vi "ReadWrite.vi"(4 "read":bool=TRUE, 5 "delay before read (ms)":u32=50, 6 "error in":errorcluster, 7 "write":bool=TRUE, 8 "string to write":string="*IDN?\r\n", 9 "VISA  name in":refnum<visa-resource-name>) -> (0 "error out":errorcluster, 1 "bytes to read":u32, 2 "read string":string, 3 "VISA out":refnum<visa-resource-name>)   [LabVIEW 2017]
doc: "The Basic Serial Read and Write example performs a Serial Port Read, a Serial Port Write, or a combination of these actions. The user selects the actions (read or write) on the front panel. If both are selected, the VI will write the data first, read data, and then close the VISA session that is opened to the port. This VI will wait until the specified number of bytes is received at the port. Only the number of bytes specified will be read.\n\nINSTRUCTIONS:\n1) Select the serial resource and configuration parameters (baud rate, data bits, parity, stop bits, flow control).\n2) Select the operations to be performed. \n3) Connect the serial port to your device. If no device is available, perform a loopback test by doing one of the following. Short pins 2 and 3 on a RS-232 cable or short pin 4 to pin 8 and pin 5 to pin 9 on a RS-485/422 cable. \n4) Run the VI to see the data read. (The \"read string\" will match the \"string to write\" if a loopback test was performed.)\n\nNote: The parameters set for the serial port must match the parameters of the connected instrument or device. In this example, the bytes to read parameter specifies the number of bytes that the serial port reads. If there were more bytes at the port than the number specified in bytes to read, those bytes would not be read. Also, if you specify to read more bytes than the number of bytes actually read, you might receive a timeout error message.\n\nOn the block diagram, the Configure Serial Port VI sets the configuration parameters. The front panel displays the controls used to configure the basic parameters, such as baud rate, data bits, and parity. Constants configure the other parameters the user probably does not need set. After the VISA Configure Serial Port VI opens the VISA session and configures the port, the VI passes the VISA resource name to other VIs that perform operations on that VISA resource. The VISA Write function sends a command to the serial device and the VISA Read function returns data based on the command. The VISA Close function then closes the reference to the serial device. It is important to close the reference; otherwise communication through with that port through protocols other than VISA might not be possible."
panel:
  out "bytes read":u32
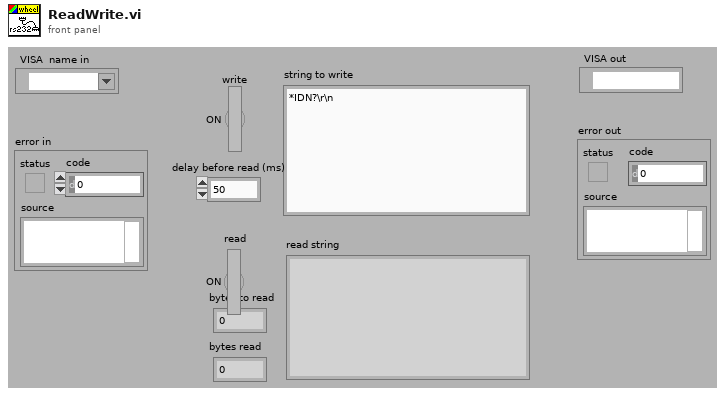
[diagram p1: front panel]
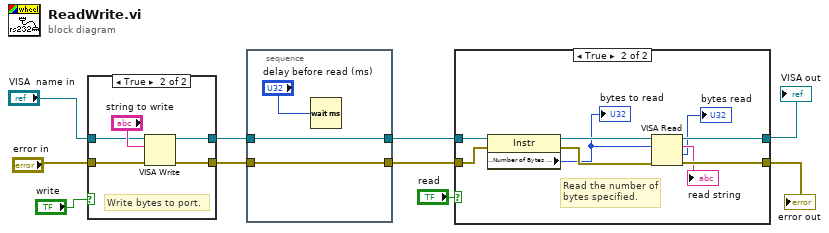
[diagram p0: block diagram]
diagram:
  n1 = case shown="True" "write" {
    tunnel: [w12 w17] -> w6
    tunnel: "VISA  name in" -> [w11 w15]
    tunnel: "error in" -> [w12 w14]
    tunnel: [w11 w13] -> w4
    frame False {
    }
    frame True {
      # "Write bytes to port."
      n2 = VISA Write(VISA resource name=w15, write buffer="string to write", error in (no error)=w14) -> (VISA resource name out=w13:refnum<visa-resource-name>, error out=w17:errorcluster)  [unwired: 1 out]
    }
  }
  n3 = stacked-sequence {
    tunnel: w6 -> [w20]
    tunnel: [w20] -> w5
    tunnel: w4 -> [w19]
    tunnel: [w19] -> w3
    frame #0 {
      n4 = Wait (ms)(milliseconds to wait="delay before read (ms)") -> ()  [unwired: 1 out]
    }
  }
  n5 = case shown="True" "read" {
    tunnel: w5 -> [w22 w27]
    tunnel: [w22 w31] -> w10
    tunnel: [w21 w30] -> w9
    tunnel: w3 -> [w21 w29]
    frame False {
    }
    frame True {
      # "Read the number of bytes specified."
      n6 = property class="Instr"(reference=w29, error in=w27) -> (reference out=w28:refnum<visa-resource-name>, error out=w26:errorcluster, "Serial Settings:Number of Bytes at Serial Port"=w24:u32)
      "bytes to read" <- w24
      n7 = VISA Read(VISA resource name=w28, byte count=w24, error in (no error)=w26) -> (VISA resource name out=w30:refnum<visa-resource-name>, read buffer=→"read string":string, return count=→"bytes read":u32, error out=w31:errorcluster)
    }
  }
  "error out" <- w10
  "VISA out" <- w9
